vi "TVA_cmd_LMS(SubVI).vi"(4 "t [s]":dbl, 6 "Sim_running":bool, 10 "TVA_yaw":dbl, 11 "TVA_pitch":dbl) -> (2 "TVA_yaw_LMS":dbl, 3 "TVA_pitch_LMS":dbl)   [LabVIEW 2017]
uses:
  <vilib>/Analysis/_algsub.llb/Real PseudoInverse Matrix.vi
  <vilib>/Analysis/baseanly.llb/Real A x B.vi
  <vilib>/Analysis/Matrix/Numeric/Conversions/Array To Matrix - RA.vi
  <vilib>/Analysis/Matrix/Numeric/Conversions/Array To Matrix - RA2.vi
  <vilib>/Analysis/Matrix/Numeric/Conversions/Matrix To Array - RM.vi
  <vilib>/Analysis/Matrix/NI_Matrix.lvlib
  <vilib>/Analysis/NI_AALPro.lvlib
  <vilib>/Analysis/NI_AALBase.lvlib
panel:
  out "yaw vec":dbl[](array[numeric])
  out "pitch vec":dbl[](array[numeric])
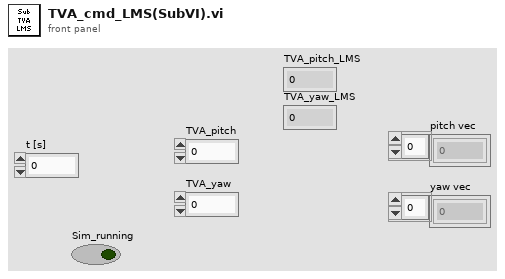
[diagram p1: front panel]
types:
  T1 = typedef "NI_Matrix.lvlib/RealMatrix.ctl" = dbl[][]
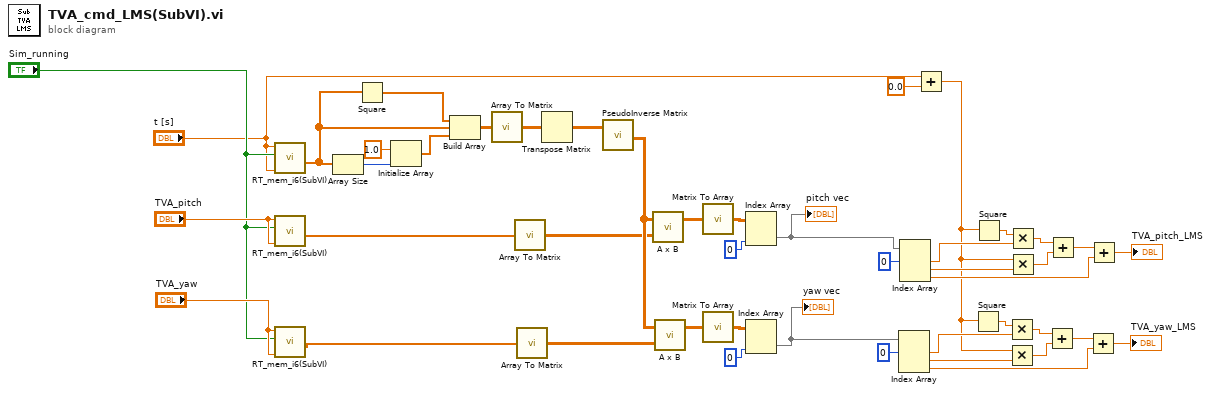
[diagram p0: block diagram]
diagram:
  n1 = call "RT_mem_i6(SubVI).vi"("Ini_val"="t [s]", "start"="Sim_running", "In"="t [s]") -> ("in_vec"=w27:dbl[])  [unwired: 7 in, 1 out]
  n2 = call "RT_mem_i6(SubVI).vi"("Ini_val"="TVA_pitch", "start"="Sim_running", "In"="TVA_pitch") -> ("in_vec"=w39:dbl[])  [unwired: 7 in, 1 out]
  n3 = call "RT_mem_i6(SubVI).vi"("Ini_val"="TVA_yaw", "start"="Sim_running", "In"="TVA_yaw") -> ("in_vec"=w36:dbl[])  [unwired: 7 in, 1 out]
  n4 = Array Size(array=w27) -> (size(s)=w24:i32)
  n5 = Square(x=w27) -> (x^2=w26:dbl[])
  n6 = Initialize Array(1.0 ("element"), w24) -> (w28:dbl[])
  n7 = Build Array(w26, w27, w28) -> (w30:dbl[][])
  n8 = call-poly <vilib>:"Array To Matrix.vi"("Real 2D Array"=w30) -> ("Real Matrix"=w29:T1)
  n9 = call-poly <vilib>:"Array To Matrix.vi"("Real 1D Array"=w39) -> ("Real Matrix (Column Vector)"=w38:T1)
  n10 = call-poly <vilib>:"Array To Matrix.vi"("Real 1D Array"=w36) -> ("Real Matrix (Column Vector)"=w32:T1)
  n11 = Transpose Matrix(1:w29) -> (0:w31:T1)
  n12 = call-poly <vilib>:"PseudoInverse Matrix.vi"("Input Matrix"=w31) -> ("PseudoInverse Matrix"=w42:T1)  [unwired: 1 in, 1 out]
  n13 = call-poly <vilib>:"A x B.vi"("B"=w38, "A"=w42) -> ("A x B"=w43:T1)  [unwired: 1 out]
  n14 = call-poly <vilib>:"A x B.vi"("B"=w32, "A"=w42) -> ("A x B"=w35:T1)  [unwired: 1 out]
  n15 = call-poly <vilib>:"Matrix To Array.vi"("Real Matrix"=w43) -> ("Real 2D Array"=w41:dbl[][])
  n16 = call-poly <vilib>:"Matrix To Array.vi"("Real Matrix"=w35) -> ("Real 2D Array"=w33:dbl[][])
  n17 = Index Array(array=w41, index (col)=0 ("index (row)")) -> (element=w6:dbl[])  [unwired: 1 in]
  "pitch vec" <- w6
  n18 = Index Array(array=w33, index (col)=0 ("index (row)")) -> (element=w7:dbl[])  [unwired: 1 in]
  "yaw vec" <- w7
  n19 = Index Array(array=w7, index #1=0 ("index")) -> (element #1=w10:dbl, element #2=w12:dbl, element #3=w15:dbl)  [unwired: 2 in]
  n20 = Index Array(array=w6, index #1=0 ("index")) -> (element #1=w21:dbl, element #2=w19:dbl, element #3=w16:dbl)  [unwired: 2 in]
  n21 = Add(x="t [s]", y=0.0) -> (x+y=w5:dbl)
  n22 = Square(x=w5) -> (x^2=w9:dbl)
  n23 = Square(x=w5) -> (x^2=w22:dbl)
  n24 = Multiply(x=w9, y=w10) -> (x*y=w11:dbl)
  n25 = Multiply(x=w5, y=w12) -> (x*y=w13:dbl)
  n26 = Multiply(x=w22, y=w21) -> (x*y=w20:dbl)
  n27 = Multiply(x=w5, y=w19) -> (x*y=w18:dbl)
  n28 = Add(x=w11, y=w13) -> (x+y=w14:dbl)
  n29 = Add(x=w20, y=w18) -> (x+y=w17:dbl)
  n30 = Add(x=w14, y=w15) -> (x+y=→"TVA_yaw_LMS":dbl)
  n31 = Add(x=w17, y=w16) -> (x+y=→"TVA_pitch_LMS":dbl)
